vi "MissingNIComponentsReportingAutoTest.vi"   [LabVIEW 2014]
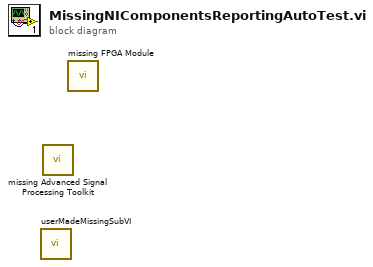
[diagram p0: block diagram]
diagram:
  n1 = call <vilib>:"userMadeMissingSubVI.vi"() -> ()  [unwired: 11 in, 1 out]
  n2 = call <vilib>:"missing Advanced Signal Processing Toolkit.vi"() -> ()  [unwired: 11 in, 1 out]
  n3 = call <vilib>:"missing FPGA Module.vi"() -> ()  [unwired: 11 in, 1 out]
